vi "2. Cast Image.vi"() -> ()   [LabVIEW 2019]
doc: "c 2020 ReMiSYS All rights reserved."
panel:
  in  "All Images? (No)":bool
  in  "Image Type":T1 items=["Grayscale (U8)", "Grayscale (I16)", "Grayscale (SGL)", "Complex (CSG)", "RGB (U32)", "HSL (U32)", "RGB (U64)", "Grayscale (U16)"]
  out "Gray Image":T2(plugin-control)
  in  "Stop (F)":bool
  out "Ori Image":T2(plugin-control)
  # "IMAQ Dispose  (Dispose All Images?)"
  # "c 2020 ReMiSYS All rights reserved."
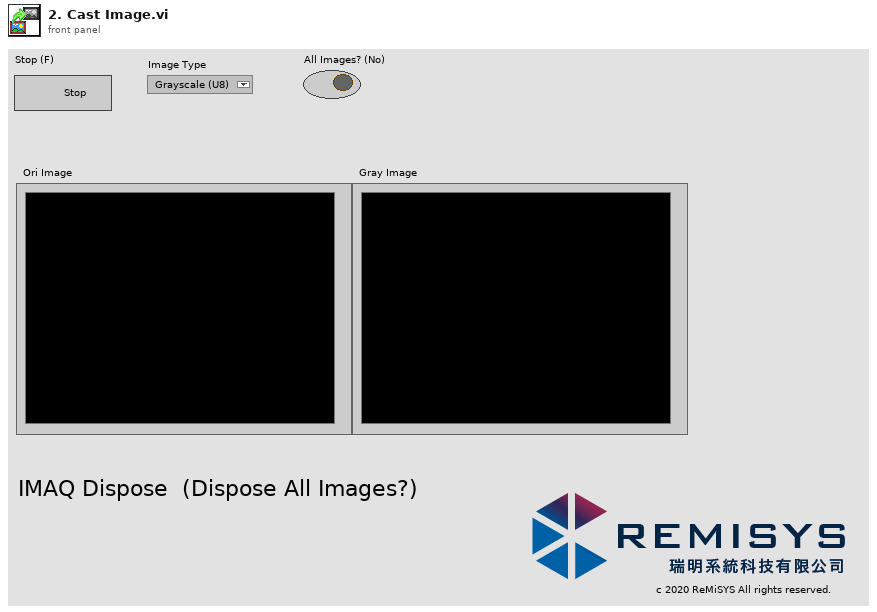
[diagram p1: front panel]
types:
  T1 = typedef "Image Type" = u32
  T2 = typedef "IMAQ Image.ctl" = refnum<image>
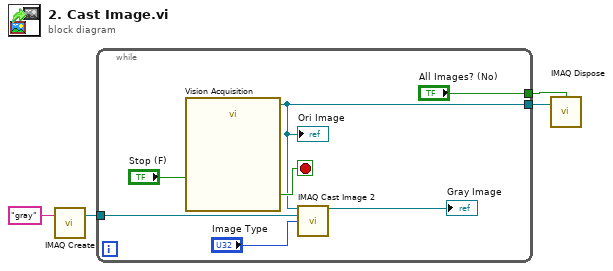
[diagram p0: block diagram]
diagram:
  n1 = call "IMAQ Create"("Image Name"="gray") -> ("New Image"=w2:T2)  [unwired: 4 in, 1 out]
  n2 = while {
    tunnel: [w8] -> w4
    tunnel: w2 -> [w9]
    tunnel: ["All Images? (No)"] -> w1
    stop <- w10 stop-if-true
    n3 = call "Vision Acquisition"("Stop (F)"="Stop (F)") -> ("Image Out"=w8:T2, "Stopped"=w10:bool)  [unwired: 24 in, 1 out]
    "Ori Image" <- w8
    n4 = call "IMAQ Cast Image 2"("Image Src"=w8, "Image Dst"=w9, "Image Type"="Image Type") -> ("Image Dst Out"=→"Gray Image":T2)  [unwired: 11 in, 1 out]
  }
  n5 = call "IMAQ Dispose"("All Images? (No)"=w1, "Image"=w4) -> ()  [unwired: 4 in, 1 out]
